vi "Test_PXF4.vi"() -> ()   [LabVIEW 2019]
uses:
  <vilib>/NI/Modbus Library/API/Master/Modbus Master.lvclass
panel:
  in  "get_ele_power":bool
  out "ele_power":dbl
  out "cj_temp":dbl
  in  "get_cj_temp":bool
  out "Output":bool
  in  "hysteresis_set":i16=1
  in  "set_hyst":bool
  out "time":timestamp format="%<%H:%M:%S\n%Y/%m/%d>T"
  out "hysteresis_get":u16
  in  "get_hyst":bool
  in  "set_SV":bool
  in  "interval":i32=1000
  in  "stop":bool
  out "SV":dbl format="%.1f"
  out "PV":dbl format="%.1f"
  in  "SV_set":dbl=70.5 format="%#_13g"
  out "error out":errorcluster
  in  "UID":u8=2
  in  "VISA":refnum<visa-resource-name>="COM7"
  # "degF"
  # "degF"
  # "degF"
  # "kWh"
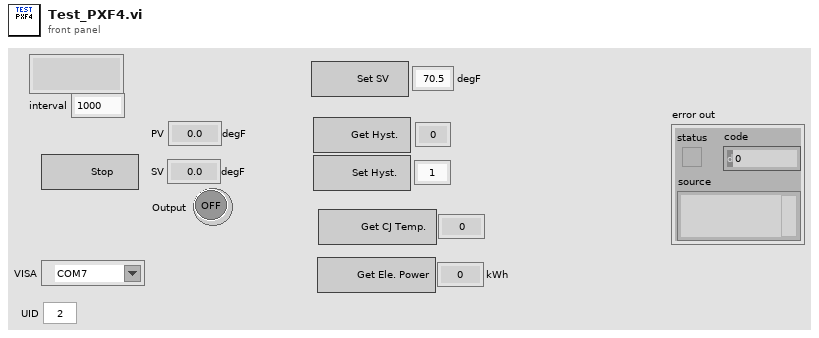
[diagram p1: front panel]
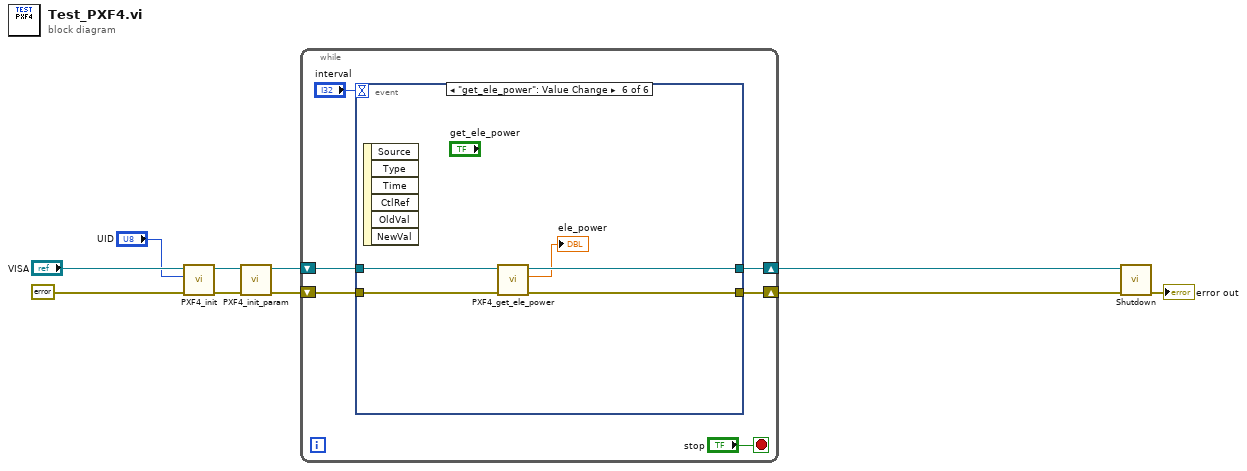
[diagram p0: block diagram]
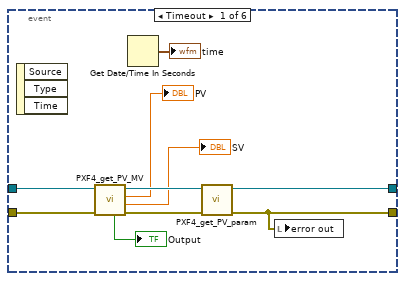
[diagram p2: hidden frame]
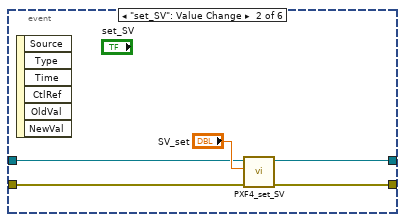
[diagram p3: hidden frame]
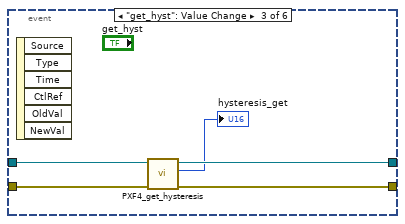
[diagram p4: hidden frame]
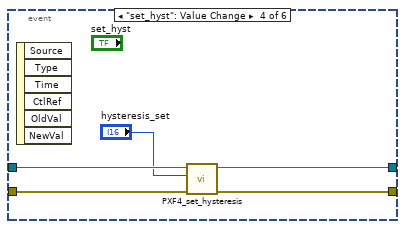
[diagram p5: hidden frame]
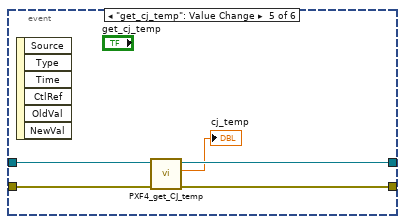
[diagram p6: hidden frame]
diagram:
  n1 = call "PXF4_init.vi"("error in"=errorcluster {"status"=FALSE, "code"=0, "source"=""}, "unit_ID"="UID", "VISA Refnum in"="VISA") -> ("error out"=w5:errorcluster, "Modbus Master out"=w6:refnum<class "Modbus Master.lvclass">)  [unwired: 7 in]
  n2 = call "PXF4_init_param.vi"("error in"=w5, "Modbus Master in"=w6) -> ("error out"=w3:errorcluster, "Modbus Master out"=w4:refnum<class "Modbus Master.lvclass">)  [unwired: 8 in]
  n3 = while {
    shift-right: [w13] -> w2
    shift-left: w4 -> [w16]
    shift-right: [w14] -> w1
    shift-left: w3 -> [w15]
    stop <- "stop" stop-if-true
    n4 = event shown="[5] \"get_ele_power\": Value Change" {
      selector: _ -> [_ _ _ _ _ _]
      dyn-events: _ -> [_ _ _ _ _ _]
      timeout: "interval" -> [_ _ _ _ _ _]
      tunnel: w16 -> [w26 w27 w36 w41 w46 w51]
      tunnel: w15 -> [w24 w28 w35 w38 w44 w49]
      tunnel: [w17 w29 w34 w39 w43 w48] -> w14
      tunnel: [w22 w30 w33 w40 w45 w50] -> w13
      event Timeout {
        n5 = event-data() -> ()  [unwired: 1 in, 3 out]
        n6 = call "PXF4_get_PV_MV.vi"("error in"=w24, "Modbus Master in"=w26) -> ("error out"=w23:errorcluster, "SV"=→"SV":dbl, "PV"=→"PV":dbl, "Modbus Master out"=w25:refnum<class "Modbus Master.lvclass">, "Output"=→"Output":bool)  [unwired: 5 in]
        n7 = Get Date/Time In Seconds() -> (seconds since 1Jan1904=→"time":timestamp)
        n8 = call "PXF4_get_PV_param.vi"("error in"=w23, "Modbus Master in"=w25) -> ("error out"=w17:errorcluster, "Modbus Master out"=w22:refnum<class "Modbus Master.lvclass">)  [unwired: 8 in]
        n9 = local write "error out"(w17) -> ()
      }
      event "set_SV": Value Change {
        n10 = event-data() -> ()  [unwired: 1 in, 6 out]
        n11 = call "PXF4_set_SV.vi"("error in"=w28, "SV"="SV_set", "Modbus Master in"=w27) -> ("error out"=w29:errorcluster, "Modbus Master out"=w30:refnum<class "Modbus Master.lvclass">)  [unwired: 7 in]
      }
      event "get_hyst": Value Change {
        n12 = event-data() -> ()  [unwired: 1 in, 6 out]
        n13 = call "PXF4_get_hysteresis.vi"("error in"=w35, "Modbus Master in"=w36) -> ("error out"=w34:errorcluster, "hysteresis"=→"hysteresis_get":i16, "Modbus Master out"=w33:refnum<class "Modbus Master.lvclass">)  [unwired: 7 in]
      }
      event "set_hyst": Value Change {
        n14 = event-data() -> ()  [unwired: 1 in, 6 out]
        n15 = call "PXF4_set_hysteresis.vi"("error in"=w38, "hysteresis"="hysteresis_set", "Modbus Master in"=w41) -> ("error out"=w39:errorcluster, "Modbus Master out"=w40:refnum<class "Modbus Master.lvclass">)  [unwired: 7 in]
      }
      event "get_cj_temp": Value Change {
        n16 = event-data() -> ()  [unwired: 1 in, 6 out]
        n17 = call "PXF4_get_CJ_temp.vi"("error in"=w44, "Modbus Master in"=w46) -> ("error out"=w43:errorcluster, "degF"=→"cj_temp":dbl, "Modbus Master out"=w45:refnum<class "Modbus Master.lvclass">)  [unwired: 7 in]
      }
      event "get_ele_power": Value Change {
        n18 = event-data() -> ()  [unwired: 1 in, 6 out]
        n19 = call "PXF4_get_ele_power.vi"("error in"=w49, "Modbus Master in"=w51) -> ("error out"=w48:errorcluster, "kWh"=→"ele_power":dbl, "Modbus Master out"=w50:refnum<class "Modbus Master.lvclass">)  [unwired: 7 in]
      }
    }
  }
  n20 = call-dynamic "Shutdown.vi"("error in"=w1, "Modbus master in"=w2) -> ("error out"=→"error out":errorcluster)  [unwired: 9 in]
